vi "PushMFC.vi"(6 "StartTime":timestamp, 8 "MFC Set 2":refnum<vi>, 11 "Array":string[](array[string])) -> (0 "Current Time":dbl, 1 "Boolean":bool, 3 "Enqueue":string)   [LabVIEW 2019, in "Scripts.lvclass"]
uses:
  Scripts.lvclass
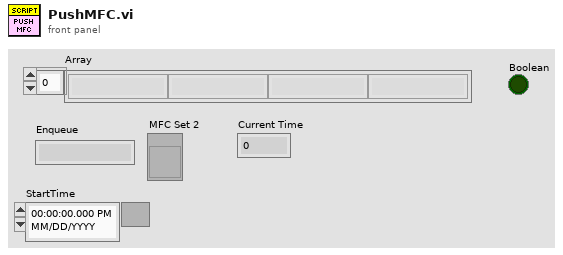
[diagram p1: front panel]
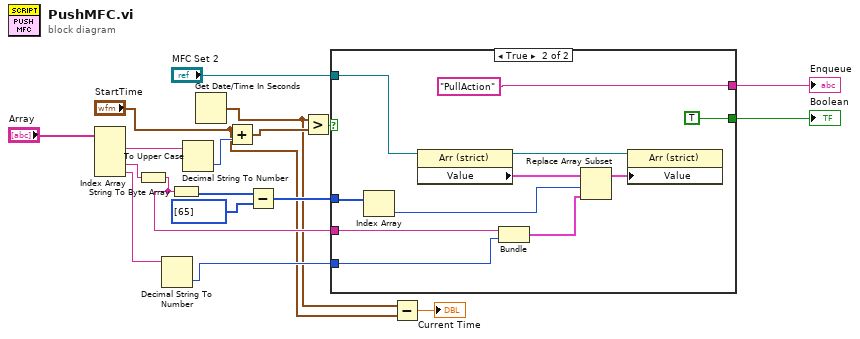
[diagram p0: block diagram]
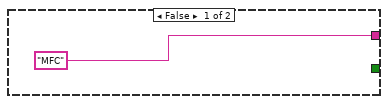
[diagram p2: hidden frame]
diagram:
  n1 = Index Array(array="Array") -> (element #1=w17:string, element #3=w7:string, element #4=w13:string)  [unwired: 4 in, 1 out]
  n2 = To Upper Case(1:w7) -> (0:w5:string)
  n3 = Decimal String To Number(string=w13) -> (number=w8:i32)  [unwired: 2 in, 1 out]
  n4 = String To Byte Array(string=w5) -> (unsigned byte array=w11:u8[])
  n5 = Decimal String To Number(string=w17) -> (number=w16:i32)  [unwired: 2 in, 1 out]
  n6 = Get Date/Time In Seconds() -> (seconds since 1Jan1904=w2:timestamp)
  n7 = Add(x="StartTime", y=w16) -> (x+y=w4:timestamp)
  n8 = Subtract(x=w11, y=u8[] [65]) -> (x-y=w9:u8[])
  n9 = Greater?(x=w2, y=w4) -> (0:w15:bool)
  n10 = case shown="True" w15 {
    tunnel: ["MFC" ("element") "PullAction" ("element")] -> w14
    tunnel: "MFC Set 2" -> [_ w29]
    tunnel: [_ TRUE] -> w12
    tunnel: w9 -> [_ w26]
    tunnel: w8 -> [_ w22]
    tunnel: w5 -> [_ w23]
    frame False {
    }
    frame True {
      n11 = Index Array(array=w26) -> (element=w24:u8)  [unwired: 1 in]
      n12 = property class="Arr (strict)"(reference=w29) -> (reference out=w28:refnum<vi>, "Value"=w25:cluster{"String":string, "MFC set":dbl}[])  [unwired: 1 in, 1 out]
      n13 = Bundle(w23, w22) -> (w21:cluster{string, i32})  [unwired: 1 in]
      n14 = Replace Array Subset(array=w25, new element=w21, index=w24) -> (w20:cluster{"String":string, "MFC set":dbl}[])
      n15 = property class="Arr (strict)"(reference=w28, "Value"=w20) -> ()  [unwired: 1 in, 2 out]
    }
  }
  "Enqueue" <- w14
  "Boolean" <- w12
  n16 = Subtract(x=w2, y="StartTime") -> (x-y=→"Current Time":dbl)
